vi "SetRunlevelForUser.vi"(8 "error in (no error)":errorcluster, 11 "LoginName":string) -> (0 "error out":errorcluster, 3 "Logon Success":bool)   [LabVIEW 2019]
uses:
  <vilib>/regexp/Match Regular Expression.xnode
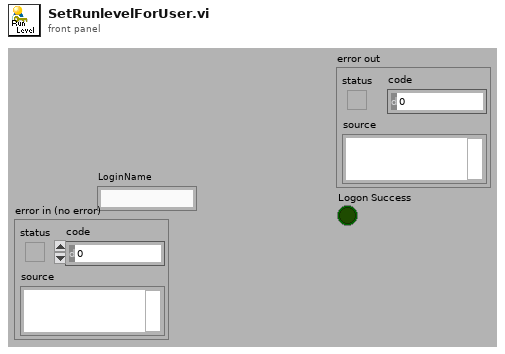
[diagram p1: front panel]
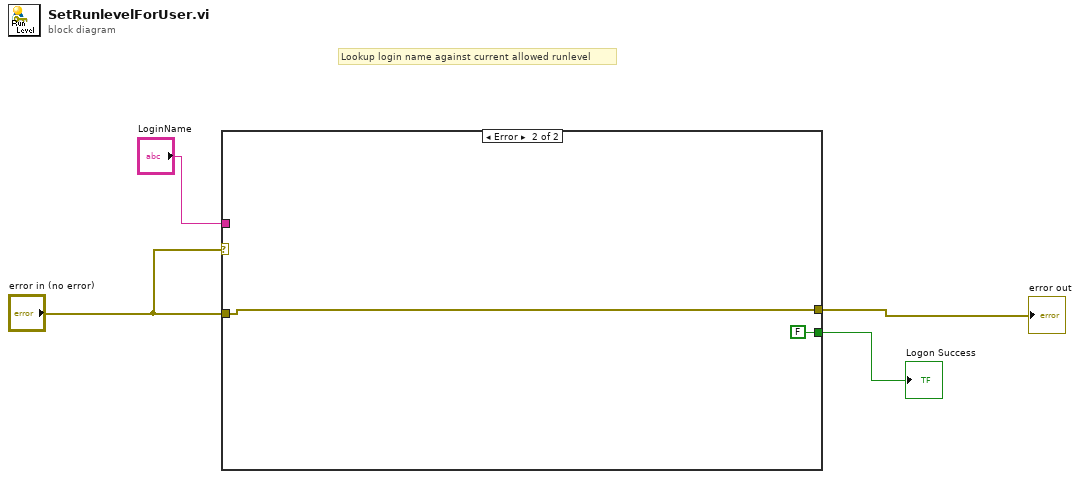
[diagram p0: block diagram]
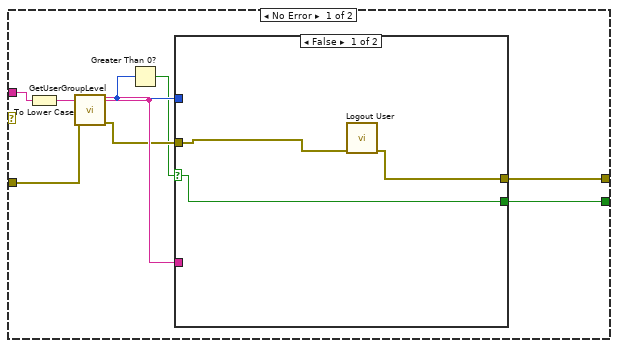
[diagram p2: hidden frame]
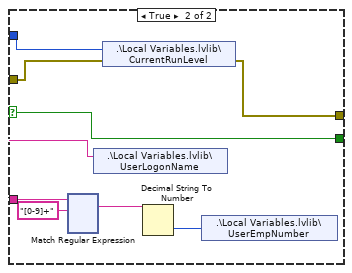
[diagram p3: hidden frame]
diagram:
  # "Lookup login name against current allowed runlevel"
  n1 = case shown="Error" "error in (no error)" {
    tunnel: "LoginName" -> [w12 _]
    tunnel: [w6 w139] -> w3
    tunnel: "error in (no error)" -> [w11 w139]
    tunnel: [w5 FALSE] -> w1
    frame No Error {
      n2 = To Lower Case(string=w12) -> (all lower case string=w10:string)
      n3 = call "GetUserGroupLevel.vi"("error in (no error)"=w11, "user"=w10) -> ("error out"=w8:errorcluster, "user level"=w9:i32)  [unwired: 8 in]
      n4 = Greater Than 0?(x=w9) -> (x > 0?=w7:bool)
      n5 = case shown="False" w7 {
        selector: w7 -> [w13 w16]
        tunnel: w10 -> [_ w20]
        tunnel: w9 -> [_ w19]
        tunnel: w8 -> [w15 w18]
        tunnel: [w14 w17] -> w6
        tunnel: [w13 w16] -> w5
        frame False {
          n6 = call "Logout User.vi"("error in (no error)"=w15) -> ("error out"=w14:errorcluster)  [unwired: 10 in]
        }
        frame True {
          n7 = xnode "Match Regular Expression"("input string"=w20, "regular expression"="[0-9]+") -> ("whole match"=w22:string)  [unwired: 4 in, 4 out]
          n8 = shared-variable ".\\Local Variables.lvlib\\UserLogonName"(w20) -> ()  [unwired: 1 in, 1 out]
          n9 = shared-variable ".\\Local Variables.lvlib\\CurrentRunLevel"(w19, error in=w18) -> (error out=w17:errorcluster)
          n10 = Decimal String To Number(string=w22) -> (number=w21:i32)  [unwired: 2 in, 1 out]
          n11 = shared-variable ".\\Local Variables.lvlib\\UserEmpNumber"(w21) -> ()  [unwired: 1 in, 1 out]
        }
      }
    }
    frame Error {
    }
  }
  "error out" <- w3
  "Logon Success" <- w1
